vi "DecodeRecordLine.vi"(8 "error in (no error)":errorcluster, 11 "Record Line":string) -> (0 "error out":errorcluster, 3 "Record Line info":T1)   [LabVIEW 2012]
doc: "Decodes .hea file first line that contains record info."
uses:
  #TD_RecordLineInfo.ctl
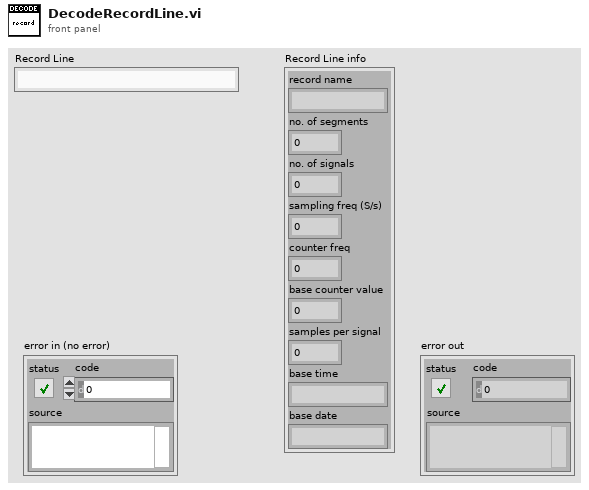
[diagram p1: front panel]
types:
  T1 = typedef "#TD_RecordLineInfo.ctl" = cluster{"record name":string, "no. of segments":i32, "no. of signals":i32, "sampling freq (S/s)":dbl, "counter freq":dbl, "base counter value":dbl, "samples per signal":i32, "base time":string, "base date":string}
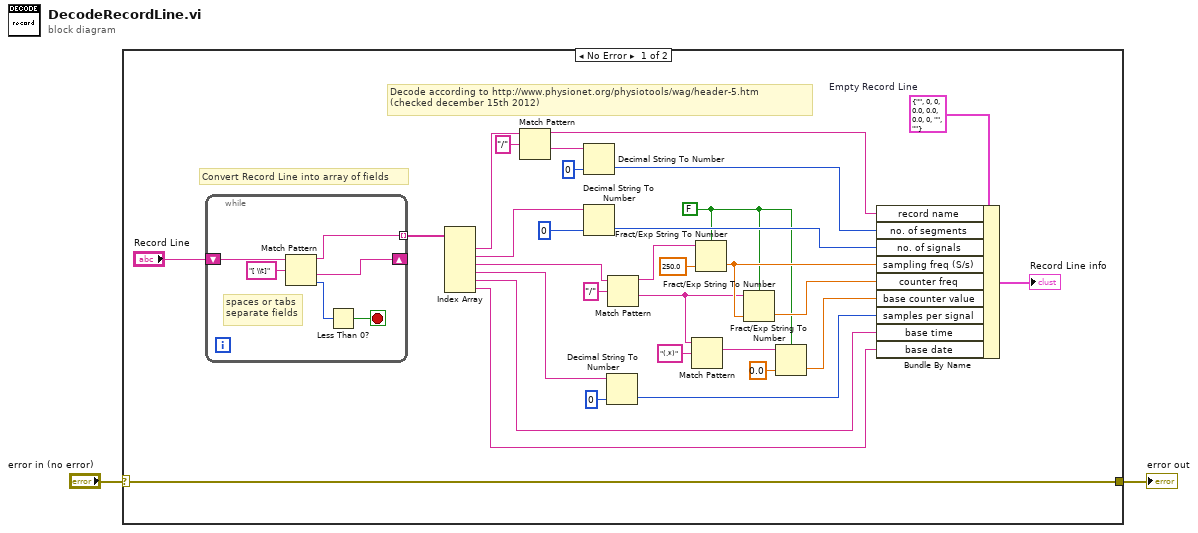
[diagram p0: block diagram]
diagram:
  n1 = case shown="No Error" "error in (no error)" {
    selector: "error in (no error)" -> [w5 w40]
    tunnel: [w5 w40] -> w1
    frame No Error {
      w4 = FALSE ("use system decimal point (T)")
      w22 = T1 {"record name"="", "no. of segments"=0, "no. of signals"=0, "sampling freq (S/s)"=0.0, "counter freq"=0.0, "base counter value"=0.0, "samples per signal"=0, "base time"="", "base date"=""}  # Empty Record Line
      # "Decode according to http://www.physionet.org/physiotools/wag/header-5.htm\n(checked december 15th 2012)"
      # "Convert Record Line into array of fields"
      n2 = while {
        shift-right: [w35] -> _
        shift-left: "Record Line" -> [w39]
        tunnel: [w34] -> w6 mode=indexing
        stop <- w37 stop-if-true
        # "spaces or tabs\nseparate fields"
        n3 = Match Pattern(string=w39, regular expression="[ \\t]") -> (before substring=w34:string, after substring=w35:string, offset past match=w38:i32)  [unwired: 1 in, 1 out]
        n4 = Less Than 0?(x=w38) -> (x < 0?=w37:bool)
      }
      n5 = Index Array(array=w6) -> (element #1=w7:string, element #2=w10:string, element #3=w16:string, element #4=w20:string, element #5=w31:string, element #6=w32:string)  [unwired: 6 in]
      n6 = Match Pattern(string=w7, regular expression="/") -> (before substring=w24:string, after substring=w9:string)  [unwired: 1 in, 2 out]
      n7 = Decimal String To Number(string=w9, default (0L)=0 ("default (0 I32)")) -> (number=w25:i32)  [unwired: 1 in, 1 out]
      n8 = Decimal String To Number(string=w10, default (0L)=0 ("default (0 I32)")) -> (number=w26:i32)  [unwired: 1 in, 1 out]
      n9 = Decimal String To Number(string=w20, default (0L)=0 ("default (0 I32)")) -> (number=w30:i32)  [unwired: 1 in, 1 out]
      n10 = Match Pattern(string=w16, regular expression="/") -> (before substring=w12:string, after substring=w17:string)  [unwired: 1 in, 2 out]
      n11 = Match Pattern(string=w17, regular expression="(.*)") -> (match substring=w18:string)  [unwired: 1 in, 3 out]
      n12 = Fract/Exp String To Number(use system decimal point (T)=w4, string=w12, default (0 dbl)=250.0 ("default (0 DBL)")) -> (number=w27:dbl)  [unwired: 1 in, 1 out]
      n13 = Fract/Exp String To Number(use system decimal point (T)=w4, string=w17, default (0 dbl)=w27) -> (number=w28:dbl)  [unwired: 1 in, 1 out]
      n14 = Fract/Exp String To Number(use system decimal point (T)=w4, string=w18, default (0 dbl)=0.0 ("default (0 DBL)")) -> (number=w29:dbl)  [unwired: 1 in, 1 out]
      n15 = Bundle By Name(cluster=w22, "record name"=w24, "no. of segments"=w25, "no. of signals"=w26, "sampling freq (S/s)"=w27, "counter freq"=w28, "base counter value"=w29, "samples per signal"=w30, "base time"=w31, "base date"=w32) -> (→"Record Line info":T1)
    }
    frame Error {
    }
  }
  "error out" <- w1
